vi "Ramp-or-stay.vi"(1 "Array in":dbl[][](array[numeric]), 2 "Slow AO Array":T1 {"Duration, Gain, NewVal" format="%#_3g"}, 3 "Voltage limit for 6723":dbl=10.0 format="%#_13g", 4 "Array 2":i32[](array[numeric])) -> (0 "Array":dbl[][](array[numeric]))   [LabVIEW 2018]
uses:
  ParameterSubCluster.ctl
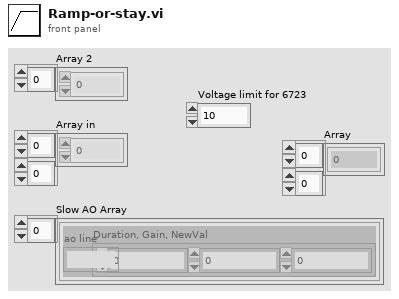
[diagram p1: front panel]
types:
  T1 = typedef "ParameterSubCluster.ctl" = cluster{"ao line":string, "Duration, Gain, NewVal":dbl[]}[]
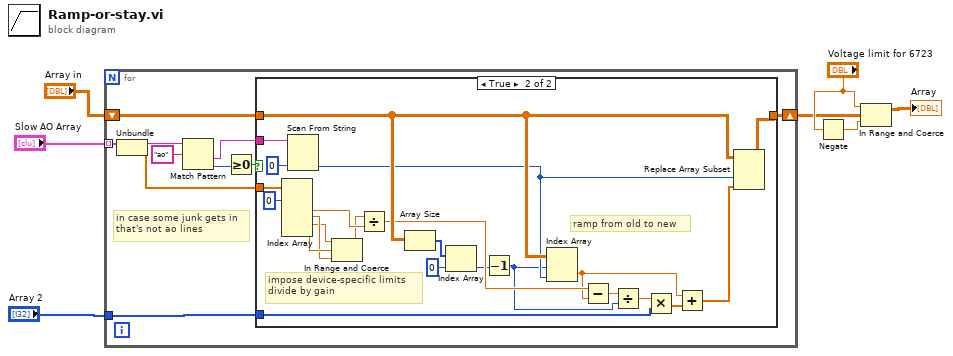
[diagram p0: block diagram]
diagram:
  n1 = for {
    tunnel: "Slow AO Array" -> [w17] mode=indexing
    tunnel: "Array 2" -> [w9]
    shift-right: [w8] -> w4
    shift-left: "Array in" -> [w11]
    # "in case some junk gets in\nthat's not ao lines"
    n2 = Unbundle(w17) -> ("ao line"=w15:string, "Duration, Gain, NewVal"=w16:dbl[])
    n3 = Match Pattern(string=w15, regular expression="ao") -> (after substring=w10:string, offset past match=w13:i32)  [unwired: 1 in, 2 out]
    n4 = Greater Or Equal To 0?(x=w13) -> (x >= 0?=w12:bool)
    n5 = case shown="True" w12 {
      tunnel: w16 -> [_ w41]
      tunnel: w11 -> [w18 w36]
      tunnel: w10 -> [_ w39]
      tunnel: w9 -> [_ w37]
      tunnel: [w18 w33] -> w8
      frame False {
      }
      frame True {
        # "ramp from old to new"
        # "impose device-specific limits\ndivide by gain"
        n6 = Index Array(array=w41, index #1=0 ("index")) -> (element #2=w40:dbl, element #3=w20:dbl, element #4=w19:dbl, element #5=w21:dbl)  [unwired: 4 in, 1 out]
        n7 = Scan From String(input string=w39, default 1=0) -> (output 1=w35:i32)  [unwired: 3 in, 3 out]
        n8 = In Range and Coerce(upper limit=w19, x=w21, lower limit=w20) -> (coerced(x)=w22:dbl)  [unwired: 1 out]
        n9 = Divide(x=w22, y=w40) -> (x/y=w34:dbl)
        n10 = Array Size(array=w36) -> (size(s)=w24:i32[])
        n11 = Index Array(array=w24, index=0) -> (element=w26:i32)
        n12 = Decrement(x=w26) -> (x-1=w31:i32)
        n13 = Index Array(array=w36, index (row)=w31, index (col)=w35) -> (element=w29:dbl)
        n14 = Subtract(x=w34, y=w29) -> (x-y=w23:dbl)
        n15 = Divide(x=w23, y=w31) -> (x/y=w27:dbl)
        n16 = Multiply(x=w27, y=w37) -> (x*y=w28:dbl[])
        n17 = Add(x=w29, y=w28) -> (x+y=w30:dbl[])
        n18 = Replace Array Subset(array=w36, new element=w30, index (col)=w35) -> (w33:dbl[][])  [unwired: 1 in]
      }
    }
  }
  n19 = Negate(x="Voltage limit for 6723") -> (-x=w6:dbl)
  n20 = In Range and Coerce(upper limit="Voltage limit for 6723", x=w4, lower limit=w6) -> (coerced(x)=→"Array":dbl[][])  [unwired: 1 out]
